vi "unitConversion.vi"(10 "Conversion Type":T1=enum."Inches -> Sensor Units", 11 "Units to Convert":dbl) -> (2 "Conversion Result":dbl)   [LabVIEW 2018]
uses:
  conversionTypeEnum.ctl
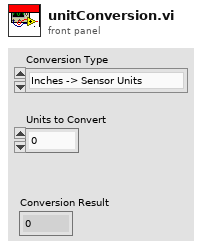
[diagram p1: front panel]
types:
  T1 = typedef "conversionTypeEnum.ctl" = enum16{"Sensor Units -> Inches", "Inches -> Sensor Units"}
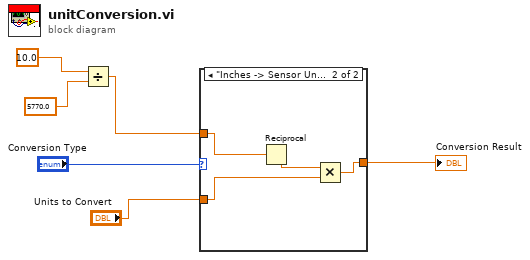
[diagram p0: block diagram]
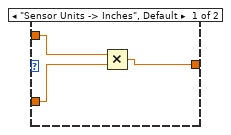
[diagram p2: hidden frame]
diagram:
  n1 = Divide(x=10.0, y=5770.0) -> (x/y=w3:dbl)
  n2 = case shown="\"Inches -> Sensor Units\"" "Conversion Type" {
    tunnel: w3 -> [w9 w13]
    tunnel: [w7 w10] -> w1
    tunnel: "Units to Convert" -> [w8 w11]
    frame "Sensor Units -> Inches", Default {
      n3 = Multiply(x=w9, y=w8) -> (x*y=w7:dbl)
    }
    frame "Inches -> Sensor Units" {
      n4 = Reciprocal(x=w13) -> (1/x=w12:dbl)
      n5 = Multiply(x=w12, y=w11) -> (x*y=w10:dbl)
    }
  }
  "Conversion Result" <- w1
